vi "Expand.vi"(8 "error in (no error)":errorcluster, 9 "CurrentLinkedNodes":refnum<data-value>[](array[refnum]), 10 "NodeToExpand in":refnum<data-value>, 11 "Graph in":refnum<class "Graph.lvclass">) -> (0 "error out":errorcluster, 1 "NodesToLinkAndExpand":refnum<data-value>[](array[refnum]), 2 "NodeToExpand out":refnum<data-value>, 3 "Graph out":refnum<class "Graph.lvclass">)   [LabVIEW 2014, in "Graph.lvlib" / "Graph.lvclass"]
doc: "Abstract method. Expands a graph's search."
uses:
  <userlib>/AdvancedDataStructures/ClassBased/Graph/Graph.lvclass
  <userlib>/AdvancedDataStructures/ClassBased/GraphNode/GraphNode.lvclass
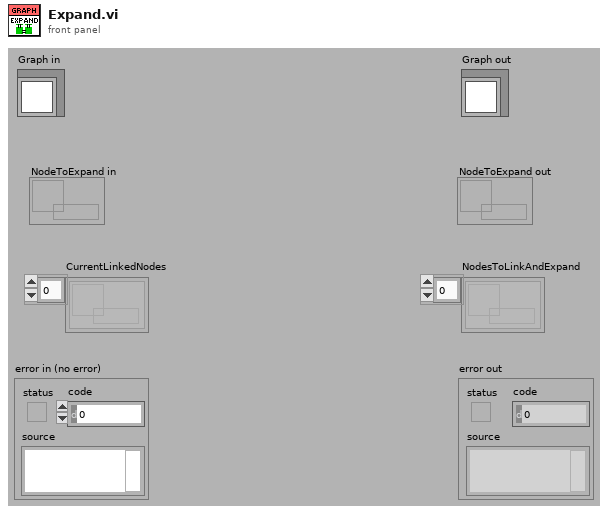
[diagram p1: front panel]
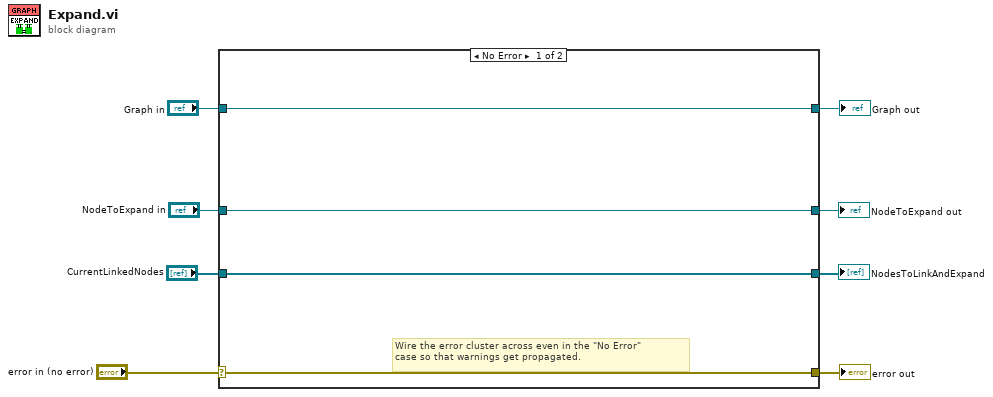
[diagram p0: block diagram]
diagram:
  n1 = case shown="No Error" "error in (no error)" {
    selector: "error in (no error)" -> [w11 w16]
    tunnel: [w11 w16] -> w7
    tunnel: [w12 w15] -> w5
    tunnel: "Graph in" -> [w12 w15]
    tunnel: [w10 w14] -> w4
    tunnel: "NodeToExpand in" -> [w10 w14]
    tunnel: "CurrentLinkedNodes" -> [w9 w13]
    tunnel: [w9 w13] -> w1
    frame No Error {
      # "Wire the error cluster across even in the \"No Error\"\ncase so that warnings get propagated."
    }
    frame Error {
    }
  }
  "error out" <- w7
  "Graph out" <- w5
  "NodeToExpand out" <- w4
  "NodesToLinkAndExpand" <- w1
